vi "KeyDown.vi"(0 "Virtual Key":u8(ring)=65, 11 "Error In":errorcluster) -> (15 "Error Out":errorcluster)   [LabVIEW 2016, in "Drona.lvlib" / "KeyboardSimulation.lvlib"]
doc: "call keybd_event drom user32.dll library to generate the key down event on desired key"
uses:
  KeyboardSimulation.lvlib
  user32.dll
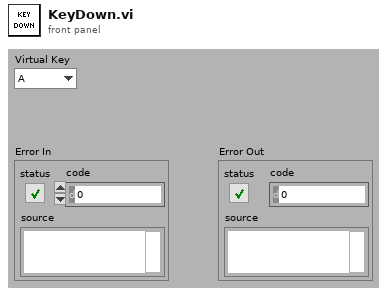
[diagram p1: front panel]
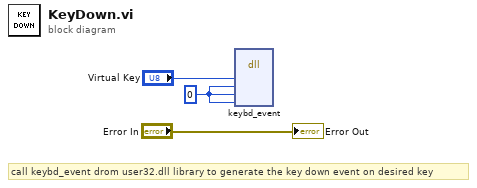
[diagram p0: block diagram]
diagram:
  w3 = u8 0 ("bScan")
  # "call keybd_event drom user32.dll library to generate the key down event on desired key"
  n1 = dll-call lib="user32.dll" fn="keybd_event"("bVk"="Virtual Key", "bScan"=w3, "dwFlags"=w3, "dwExtraInfo"=w3) -> ()  [unwired: 8 in, 2 out]
  "Error Out" <- "Error In"
